vi "DesktopDevice.vi"() -> ()   [LabVIEW 2017]
uses:
  <vilib>/addons/InsightCM/Devices/Shared/Cms/CmsAcquisition/subVIs/SimulatedConfigRefGlobal.vi
  <vilib>/addons/InsightCM/Devices/Shared/Cms/CmsAcquisition/CmsAcquisition.lvlib
  <vilib>/addons/InsightCM/Utilities/GlobalConfiguration/GlobalConfiguration.lvlib
panel:
  out "Name":string
  out "Error":string
  out "Application:Command Line Arguments":string[](array[string])
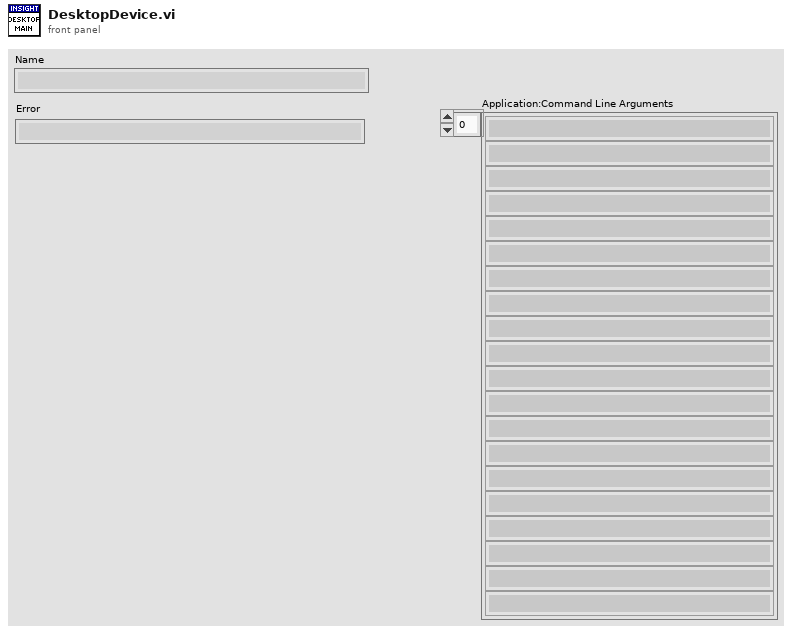
[diagram p1: front panel]
types:
  T1 = typedef "R2_Device.ctl" = cluster{"Id":string, "Name":string, "DeviceType":string, "HardwareName":string, "IpAddress":string, "HardwareInfo":T2[], "ApplicationType":string, "ApplicationVersion":string, "EquipmentIds":string[], "ConfigurationVersion":string, "State":T3, "Properties":T2[], "DataGroups":T4[], "BurstModeTrigger":T8}
  T2 = typedef "KeyValuePair.ctl" = cluster{"Key":string, "Value":string}
  T3 = typedef "DeviceState.ctl" = cluster{"Disabled":bool}
  T4 = typedef "R2_DataGroup.ctl" = cluster{"Name":string, "OperatingStates":T5[], "Properties":T2[], "EquipmentIds":string[], "AssetNodeId":string}
  T5 = typedef "OperatingState.ctl" = cluster{"Name":string, "Properties":T2[], "Triggers":T6[]}
  T6 = typedef "Trigger.ctl" = cluster{"Type":string, "Expression":string, "Conditions":T7[]}
  T7 = typedef "Condition.ctl" = cluster{"Source":string, "Type":string, "Operator":string, "CompareTo":string, "DwellSeconds":dbl}
  T8 = typedef "BurstModeTrigger.ctl" = cluster{"Trigger":T6, "SampleRate":string, "AcquisitionLength":string}
  T9 = enum32{"invalid app kind", "Development System", "Run Time System", "Student Edition", "Embedded LabVIEW", "Evaluation", "Custom"}
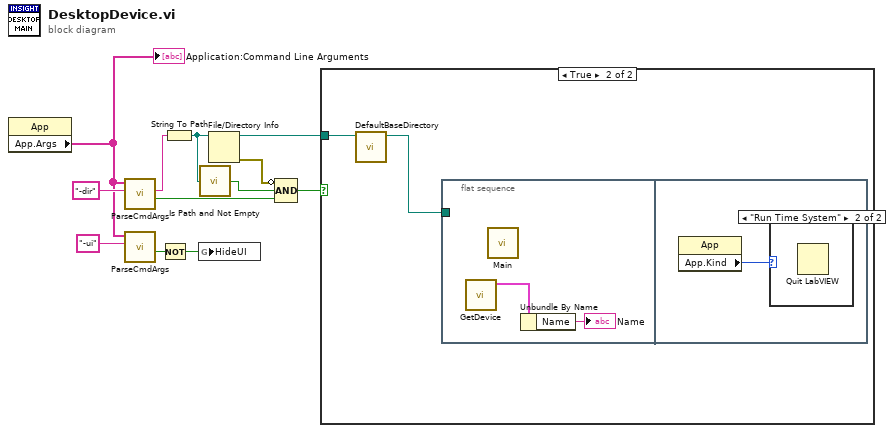
[diagram p0: block diagram]
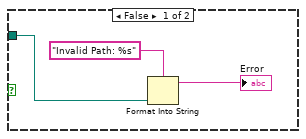
[diagram p2: hidden frame]
diagram:
  n1 = property class="App"() -> ("App.Args"=w10:string[])  [unwired: 2 in, 2 out]
  "Application:Command Line Arguments" <- w10
  n2 = call <vilib>:"ParseCmdArgs.vi"("key"="-dir", "CmdArgs"=w10) -> ("found"=w7:bool, "value"=w9:string)  [unwired: 8 in]
  n3 = call <vilib>:"ParseCmdArgs.vi"("key"="-ui", "CmdArgs"=w10) -> ("found"=w2:bool)  [unwired: 8 in, 1 out]
  n4 = Not(x=w2) -> (.not. x?=w1:bool)
  n5 = String To Path(string=w9) -> (path=w8:path)
  n6 = global write "SimulatedConfigRefGlobal.vi" "HideUI"(w1) -> ()
  n7 = call <vilib>:"Is Path and Not Empty.vi"("path"=w8) -> ("Is Path and Not Empty?"=w5:bool)  [unwired: 4 in]
  n8 = File/Directory Info(path=w8) -> (path out=w3:path, error out=w4:errorcluster)  [unwired: 1 in, 5 out]
  n9 = Compound Arithmetic op=AND(invert w4, w5, w7) -> (w6:bool)
  n10 = case shown="True" w6 {
    tunnel: w3 -> [w14 w17]
    frame False {
      n11 = Format Into String(format string="Invalid Path: %s", w14) -> (resulting string=→"Error":string)  [unwired: 2 in, 1 out]
    }
    frame True {
      n12 = call <vilib>:"DefaultBaseDirectory.vi"("base directory in"=w17) -> ("base directory"=w16:path)  [unwired: 10 in]
      n13 = flat-sequence {
        tunnel: w16 -> [_]
        frame #0 {
          n14 = call <vilib>:"GetDevice.vi"() -> ("device configuration"=w18:T1)  [unwired: 9 in, 2 out]
          n15 = call "Main.vi"() -> ()  [unwired: 12 in]
          n16 = Unbundle By Name(w18) -> ("Name"=→"Name":string)
        }
        frame #1 {
          n17 = property class="App"() -> ("App.Kind"=w20:T9)  [unwired: 2 in, 2 out]
          n18 = case shown="\"Run Time System\"" w20 {
            frame "invalid app kind", Default {
            }
            frame "Run Time System" {
              n19 = Quit LabVIEW() -> ()  [unwired: 1 in]
            }
          }
        }
      }
    }
  }
